vi "Part 1.vi"(11 "Input":string) -> (3 "Output":i64)   [LabVIEW 2021]
uses:
  <userlib>/_OpenG.lib/string/string.llb/Convert EOLs (String)__ogtk.vi
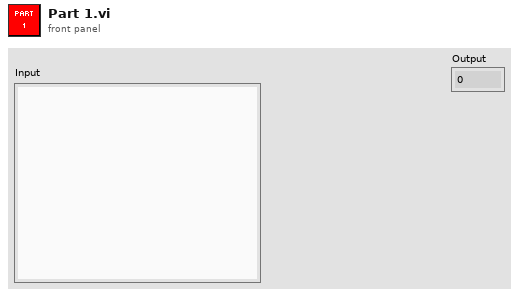
[diagram p1: front panel]
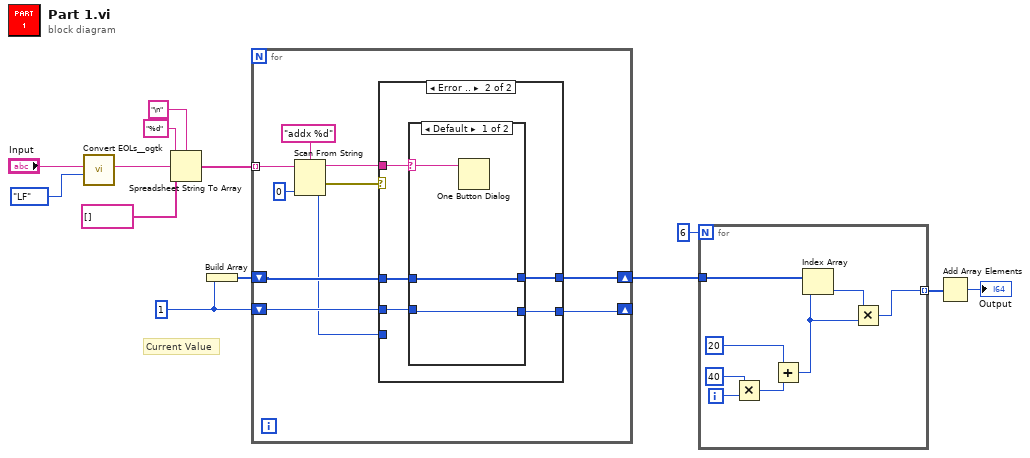
[diagram p0: block diagram]
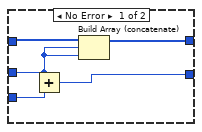
[diagram p2: hidden frame]
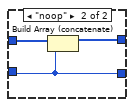
[diagram p3: hidden frame]
diagram:
  w5 = i64 1
  # "Current Value"
  n1 = call-poly <userlib>:"Convert EOLs__ogtk.vi"("Convert to:"=enum16{"CR", "LF", "CRLF"}."LF", "String in"="Input") -> ("String out"=w9:string)  [unwired: 9 in]
  n2 = Spreadsheet String To Array(delimiter (Tab)="\n", format string="%d", spreadsheet string=w9, array type (2D Dbl)=string[] []) -> (array=w7:string[])
  n3 = Build Array(w5) -> (w6:i64[])
  n4 = for {
    tunnel: w7 -> [w23] mode=indexing
    shift-right: [w18] -> w4
    shift-left: w6 -> [w20]
    shift-right: [w17] -> _
    shift-left: w5 -> [w19]
    n5 = Scan From String(format string="addx %d", input string=w23, default 1=i64 0 ("default value 1")) -> (remaining string=w21:string, error out=w22:errorcluster, output 1=w16:i64)  [unwired: 2 in, 1 out]
    n6 = case shown="Error .." w22 {
      tunnel: w21 -> [_ w33]
      tunnel: w20 -> [w25 w32]
      tunnel: w19 -> [w26 w31]
      tunnel: [w24 w30] -> w18
      tunnel: [w27 w29] -> w17
      tunnel: w16 -> [w28 _]
      frame No Error {
        n7 = Add(x=w26, y=w28) -> (x+y=w27:i64)
        n8 = Build Array (concatenate)(w25, w26, w26) -> (w24:i64[])
      }
      frame Error {
        n9 = case shown="Default" w33 {
          selector: w33 -> [w36 _]
          tunnel: w32 -> [w35 w39]
          tunnel: w31 -> [w34 w37]
          tunnel: [w35 w38] -> w30
          tunnel: [w34 w37] -> w29
          frame Default {
            n10 = One Button Dialog(message=w36) -> ()  [unwired: 1 in, 1 out]
          }
          frame "noop" {
            n11 = Build Array (concatenate)(w39, w37) -> (w38:i64[])
          }
        }
      }
    }
  }
  n12 = for {
    N: 6 -> [_]
    tunnel: w4 -> [w47]
    tunnel: [w45] -> w3 mode=indexing
    i -> [w42]
    n13 = Multiply(x=40, y=w42) -> (x*y=w43:i32)
    n14 = Add(x=20, y=w43) -> (x+y=w41:i32)
    n15 = Index Array(array=w47, index=w41) -> (element=w46:i64)
    n16 = Multiply(x=w46, y=w41) -> (x*y=w45:i64)
  }
  n17 = Add Array Elements(numeric array=w3) -> (sum=→"Output":i64)
